vi "_Read.vi"(8 "error in (no error)":errorcluster, 11 "Dummy in":refnum<class "Dummy.lvclass">) -> (0 "error out":errorcluster, 2 "4 Data Points":dbl[](array[numeric]), 3 "Dummy out":refnum<class "Dummy.lvclass">)   [LabVIEW 2009, in "Dummy.lvclass"]
uses:
  Dummy.lvclass
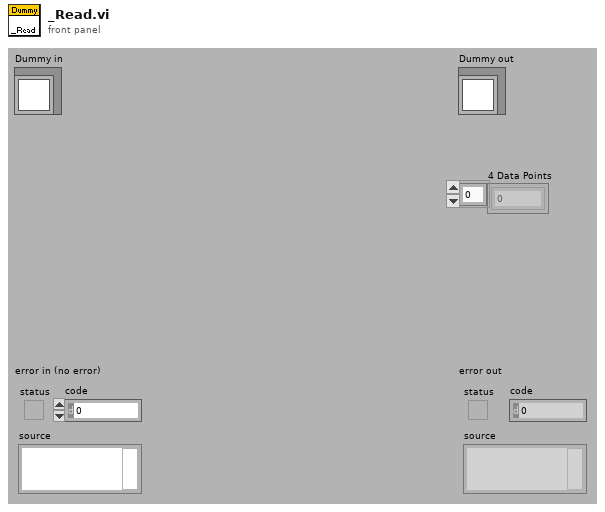
[diagram p1: front panel]
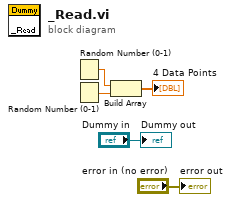
[diagram p0: block diagram]
diagram:
  n1 = Random Number (0-1)() -> (number: 0 to 1=w3:dbl)
  n2 = Random Number (0-1)() -> (number: 0 to 1=w1:dbl)
  n3 = Build Array(w3, w1) -> (→"4 Data Points":dbl[])
  "error out" <- "error in (no error)"
  "Dummy out" <- "Dummy in"
